vi "Send Self-Addressed Message.vi"(8 "error in (no error)":errorcluster, 11 "Self-Addressed Message in":refnum<class "Self-Addressed Msg.lvclass">) -> (0 "error out":errorcluster, 3 "Self-Addressed Message out":refnum<class "Self-Addressed Msg.lvclass">)   [LabVIEW 2020, in "Actor Framework.lvlib" / "Self-Addressed Msg.lvclass"]
doc: "<p>(<strong>Filename</strong>: <span class=\"dnl\">Actor Framework.lvlib:Self-Addressed Msg.lvclass:Send Self-Addressed Message.vi</span>)</p>\n\n<p>Sends a self-addressed message. You can send multiple copies to the same address by calling this VI multiple times with the same message.</p>\n\n<p>Use the <a href=\"nihelplauncher://docs/csh?context=lvcore_lvcomm_af_address_message\">Address Message</a> method to create a self-addressed message.</p>"
uses:
  Self-Addressed Msg.lvclass
  Self-Addressed Msg.lvclass/Self-Addressed Msg.ctl
  Message Enqueuer/Message Enqueuer.lvclass
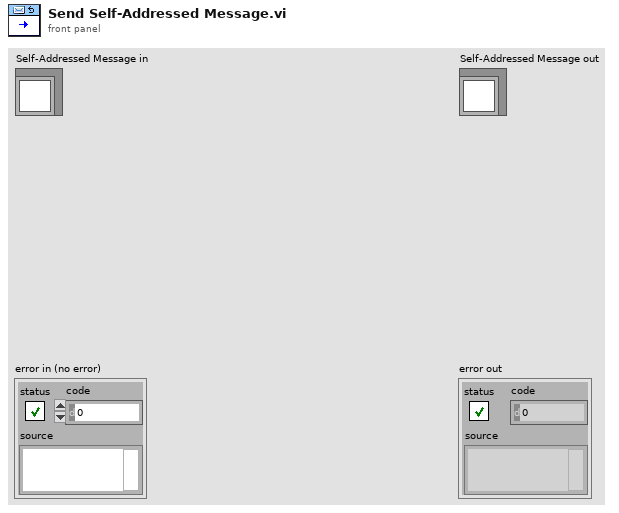
[diagram p1: front panel]
types:
  T1 = typedef "Actor Framework.lvlib/Message Enqueuer.lvclass/Message Priority.ctl" = enum16{"Low", "Normal", "High"}
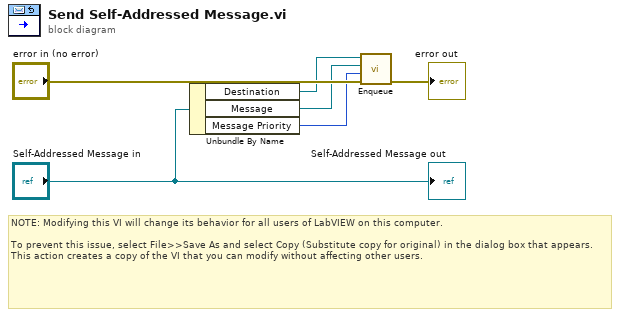
[diagram p0: block diagram]
diagram:
  # "NOTE: Modifying this VI will change its behavior for all users of LabVIEW on this computer.\n\nTo prevent this issue, select File>>Save As and select Copy (Substitute copy for original) in the dialog box that appears. This action creates a copy of the VI that you can modify without affecting other users."
  n1 = Unbundle By Name("Self-Addressed Message in") -> ("Destination"=w3:refnum<class "Message Enqueuer.lvclass">, "Message"=w2:refnum<class "Message.lvclass">, "Message Priority"=w1:T1)
  n2 = call "Enqueue.vi"("error in (no error)"="error in (no error)", "Message Priority (Normal)"=w1, "Message"=w2, "Message Enqueuer in"=w3) -> ("error out"=→"error out":errorcluster)  [unwired: 6 in, 1 out]
  "Self-Addressed Message out" <- "Self-Addressed Message in"
